vi "Get Message From Mediator.vi"(8 "error in (no error)":errorcluster caption="错误输入（无错误）", 11 "Colleague 输入":refnum<class "Colleague.lvclass"> caption="DNL_LabVIEW Object in") -> (0 "error out":errorcluster caption="错误输出", 2 "Message.lvclass":refnum<class "Message.lvclass">, 3 "Colleague 输出":refnum<class "Colleague.lvclass"> caption="DNL_LabVIEW Object out")   [LabVIEW 2011, in "Colleague.lvclass"]
uses:
  Colleague.lvclass
  Colleague.lvclass/Colleague.ctl
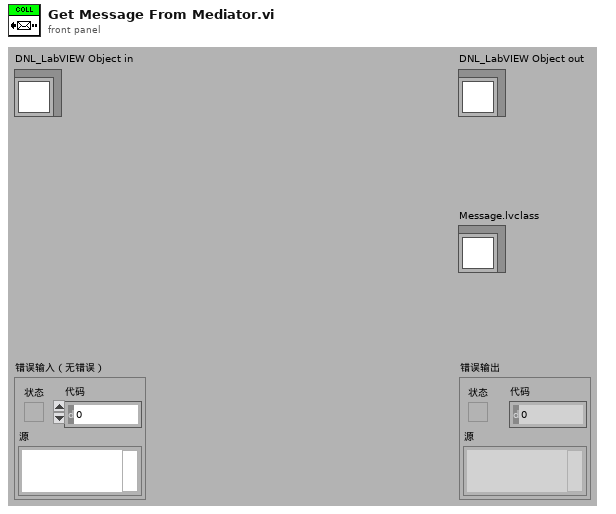
[diagram p1: front panel]
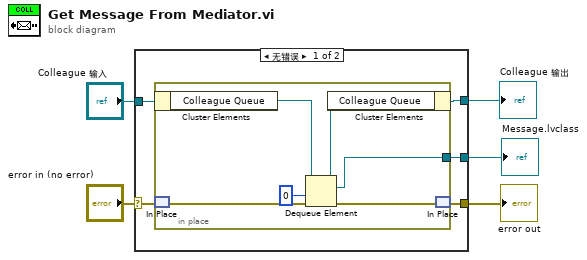
[diagram p0: block diagram]
diagram:
  n1 = case shown="无错误" "error in (no error)" {
    selector: "error in (no error)" -> [w7 w18]
    tunnel: [w6 w18] -> w4
    tunnel: [w9 w17] -> w2
    tunnel: "Colleague 输入" -> [w10 w17]
    tunnel: [w8 _] -> w1
    frame No Error {
      n2 = in-place {
        in-place-border: [w13] -> w8
        n3 = in-place-cluster #1(w10) -> ("Colleague Queue"=w15:refnum<queue>)
        n4 = in-place-match #2(w7) -> (w12:errorcluster)
        n5 = Dequeue Element(queue=w15, timeout in ms (-1)=0 ("超时毫秒(-1)"), error in (no error)=w12) -> (queue out=w14:refnum<queue>, element=w13:refnum<class "Message.lvclass">, error out=w11:errorcluster)  [unwired: 1 out]
        n6 = in-place-cluster #1("Colleague Queue"=w14) -> (w9:refnum<class "Colleague.lvclass">)
        n7 = in-place-match #2(w11) -> (w6:errorcluster)
      }
    }
    frame Error {
    }
  }
  "error out" <- w4
  "Colleague 输出" <- w2
  "Message.lvclass" <- w1
